vi "SlewRate Validity.vi"(0 "Measured Slew Rate":dbl, 11 "error in (no error)":errorcluster) -> (4 "Slew rate Out":dbl, 6 "Edge not found?":bool, 15 "error out":errorcluster)   [LabVIEW 2020, in "LDO Load Transient_AWG.lvlib"]
uses:
  LDO Load Transient_AWG.lvlib
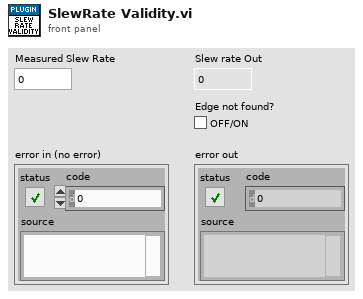
[diagram p1: front panel]
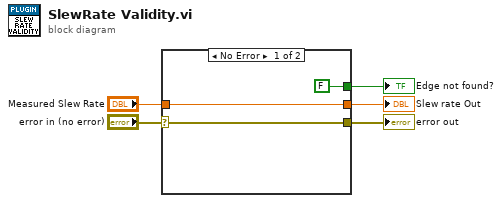
[diagram p0: block diagram]
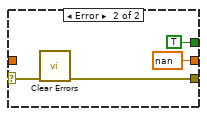
[diagram p2: hidden frame]
diagram:
  n1 = case shown="No Error" "error in (no error)" {
    selector: "error in (no error)" -> [w8 w11]
    tunnel: [w8 w10] -> w3
    tunnel: [w7 nan] -> w4
    tunnel: "Measured Slew Rate" -> [w7 _]
    tunnel: [FALSE TRUE] -> w1
    frame No Error {
    }
    frame Error {
      n2 = call <vilib>:"Clear Errors.vi"("error in (no error)"=w11) -> ("error out"=w10:errorcluster)  [unwired: 5 in, 1 out]
    }
  }
  "Slew rate Out" <- w4
  "error out" <- w3
  "Edge not found?" <- w1
